vi "Data type to datagridview string.vi"() -> (3 "String":string)   [LabVIEW 2013]
uses:
  <vilib>/NI/Tag Bus/tag/Data Type.ctl
  LabVIEWdotNetDataGrid/source/DataGridView/DataGridView.lvclass
  <vilib>/NI/Tag Bus/tag/tag descriptor.lvclass
panel:
  in  "dt":T1
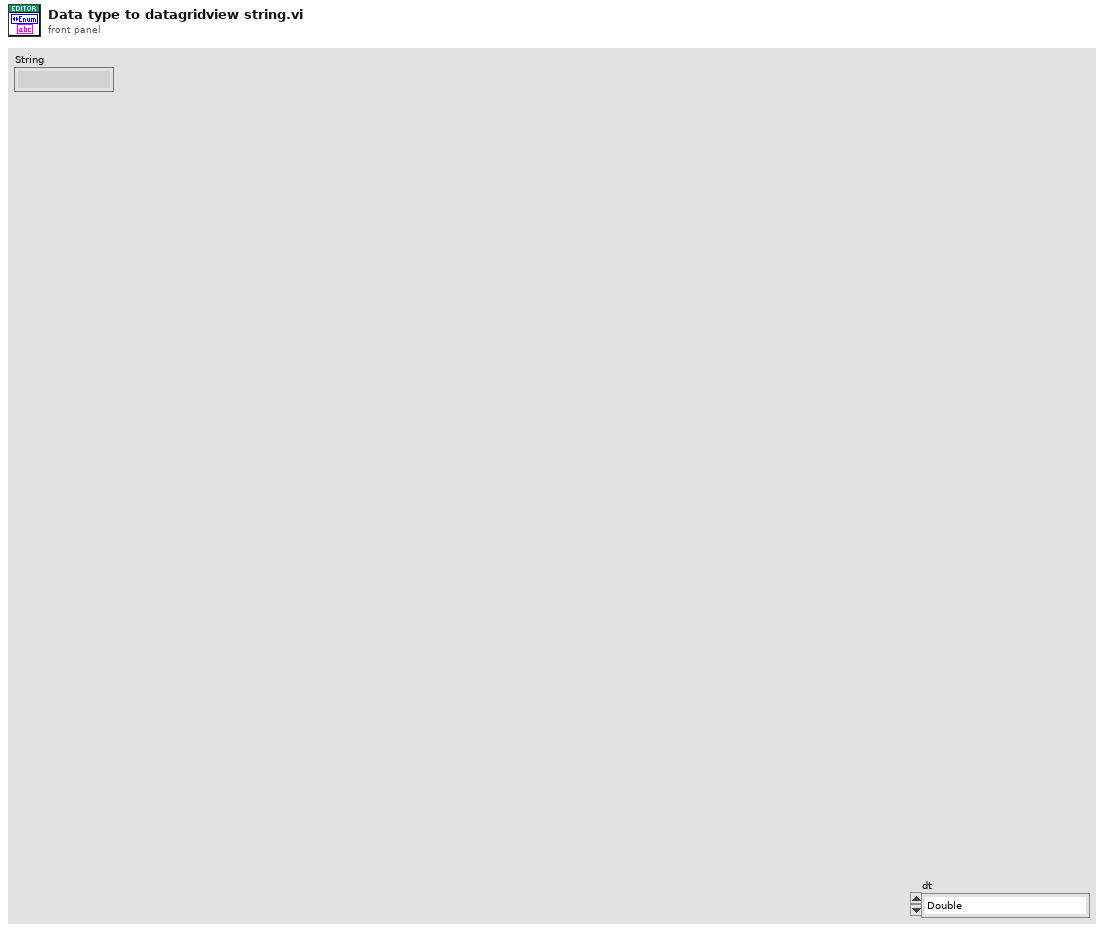
[diagram p1: front panel]
types:
  T1 = typedef "tag bus.lvlib/tag descriptor.lvclass/Data Type.ctl" = enum16{"Double", "Single", "I64", "I32", "I16", "I8", "U64", "U32", "U16", "U8", "Boolean", "String", "Array of Double", "Array of Single", "Array of I64", "Array of I32", "Array of I16", "Array of I8", "Array of U64", "Array of U32", "Array of U16", "Array of U8", "Array of Boolean", "Array of String"}
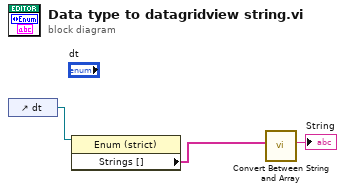
[diagram p0: block diagram]
diagram:
  n1 = control-ref of="dt"() -> (w1:refnum<vi>)
  n2 = property class="Enum (strict)"(reference=w1) -> ("Strings []"=w2:string[])  [unwired: 1 in, 2 out]
  n3 = call "Convert Between String and Array.vi"("String Array"=w2) -> ("String"=→"String":string)  [unwired: 9 in, 1 out]
